vi "TrajectoryGenerate_Make_Quintic.vi"(8 "traj_config":T6 {"End Velocity" format="%20.4f"; "StartVelocity" format="%20.4f"; "Max Acceleration" format="%20.4f"; "MaxVelocity" format="%20.4f"}, 11 "waypointPOSE":T1[](array[typedef]) {"ROTATION"."SIN" format="%13.4f"; "ROTATION"."COS" format="%13.4f"; "ROTATION"."VALUE" format="%13.4f"; "TRANSLATION"."Y" format="%14.3f"; "TRANSLATION"."X" format="%14.3f"}) -> (0 "error out":errorcluster, 3 "TRAJECTORY":T4 {"States"."POSE"."ROTATION"."SIN" format="%13.4f"; "States"."POSE"."ROTATION"."COS" format="%13.4f"; "States"."POSE"."ROTATION"."VALUE" format="%13.4f"; "States"."POSE"."TRANSLATION"."Y" format="%14.3f"; "States"."POSE"."TRANSLATION"."X" format="%14.3f"; "TotalTImeSecs" format="%20.3f"})   [LabVIEW 2019, in "Trajectory_Library.lvlib"]
doc: "Generates a trajectory from the given waypoints and config. This method uses quintic hermite splines -- therefore, all points must be represented by Pose2d objects. Continuous curvature is guaranteed in this method.\n\nParameters:\n - WaypointPose - Array of waypoints (Pose).\n - Trajectory Config - The configuration for the trajectory.\n\nReturns:\n - Trajectory -- Created trajectory data structure\n - Error Out - Returned error cluster"
uses:
  Trajectory_Library.lvlib
  TypeDef/TRANSLATION2D.ctl
  TypeDef/ROTATION2D.ctl
  TypeDef/POSE2D.ctl
  TypeDef/POSEwCURVATURE.ctl
  TypeDef/TRAJ_STATE.ctl
  TypeDef/TRAJECTORY.ctl
  TypeDef/TRAJ_CONFIG.ctl
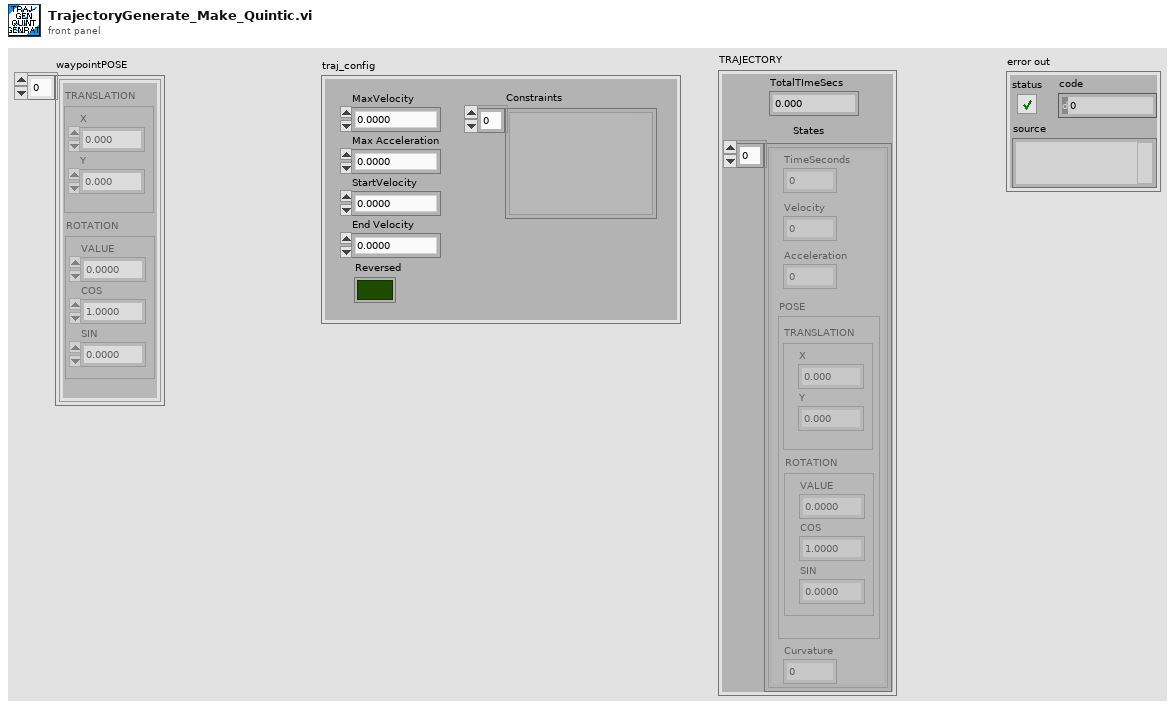
[diagram p1: front panel]
types:
  T1 = typedef "Trajectory_Library.lvlib/POSE2D.ctl" = cluster{"TRANSLATION":T2, "ROTATION":T3}
  T2 = typedef "Trajectory_Library.lvlib/TRANSLATION2D.ctl" = cluster{"X":dbl, "Y":dbl}
  T3 = typedef "Trajectory_Library.lvlib/ROTATION2D.ctl" = cluster{"VALUE":dbl, "COS":dbl, "SIN":dbl}
  T4 = typedef "Trajectory_Library.lvlib/TRAJECTORY.ctl" = cluster{"TotalTImeSecs":dbl, "States":T5[]}
  T5 = typedef "Trajectory_Library.lvlib/TRAJ_STATE.ctl" = cluster{"TimeSeconds":dbl, "Velocity":dbl, "Acceleration":dbl, "POSE":T1, "Curvature":dbl}
  T6 = typedef "Trajectory_Library.lvlib/TRAJ_CONFIG.ctl" = cluster{"MaxVelocity":dbl, "Max Acceleration":dbl, "StartVelocity":dbl, "End Velocity":dbl, "Reversed":bool, "Constraints":variant[]}
  T7 = typedef "WPILib_Math.lvlib/ROTATION2D.ctl" = cluster{"VALUE":dbl, "COS":dbl, "SIN":dbl}
  T8 = typedef "WPILib_Math.lvlib/TRANSLATION2D.ctl" = cluster{"X":dbl, "Y":dbl}
  T9 = typedef "WPILib_Math.lvlib/TRANSFORM2D.ctl" = cluster{"TRANSLATION":T8, "ROTATION":T7, "xF":bool}
  T10 = typedef "WPILib_Math.lvlib/POSE2D.ctl" = cluster{"TRANSLATION":T8, "ROTATION":T7}
  T11 = typedef "WPILib_Math.lvlib/SPLINE.ctl" = cluster{"Degree":i32, "Coefficients":T12}
  T12 = typedef "NI_Matrix.lvlib/RealMatrix.ctl" = dbl[][]
  T13 = typedef "Trajectory_Library.lvlib/POSEwCURVATURE.ctl" = cluster{"CURVATURE":dbl, "POSE":T1}
  T14 = typedef "WPILib_Math.lvlib/POSEwCURVATURE.ctl" = cluster{"CURVATURE":dbl, "POSE":T10}
  T15 = typedef "WPILib_Math.lvlib/TRAJECTORY.ctl" = cluster{"TotalTImeSecs":dbl, "States":T16[]}
  T16 = typedef "WPILib_Math.lvlib/TRAJ_STATE.ctl" = cluster{"TimeSeconds":dbl, "Velocity":dbl, "Acceleration":dbl, "POSE":T10, "Curvature":dbl}
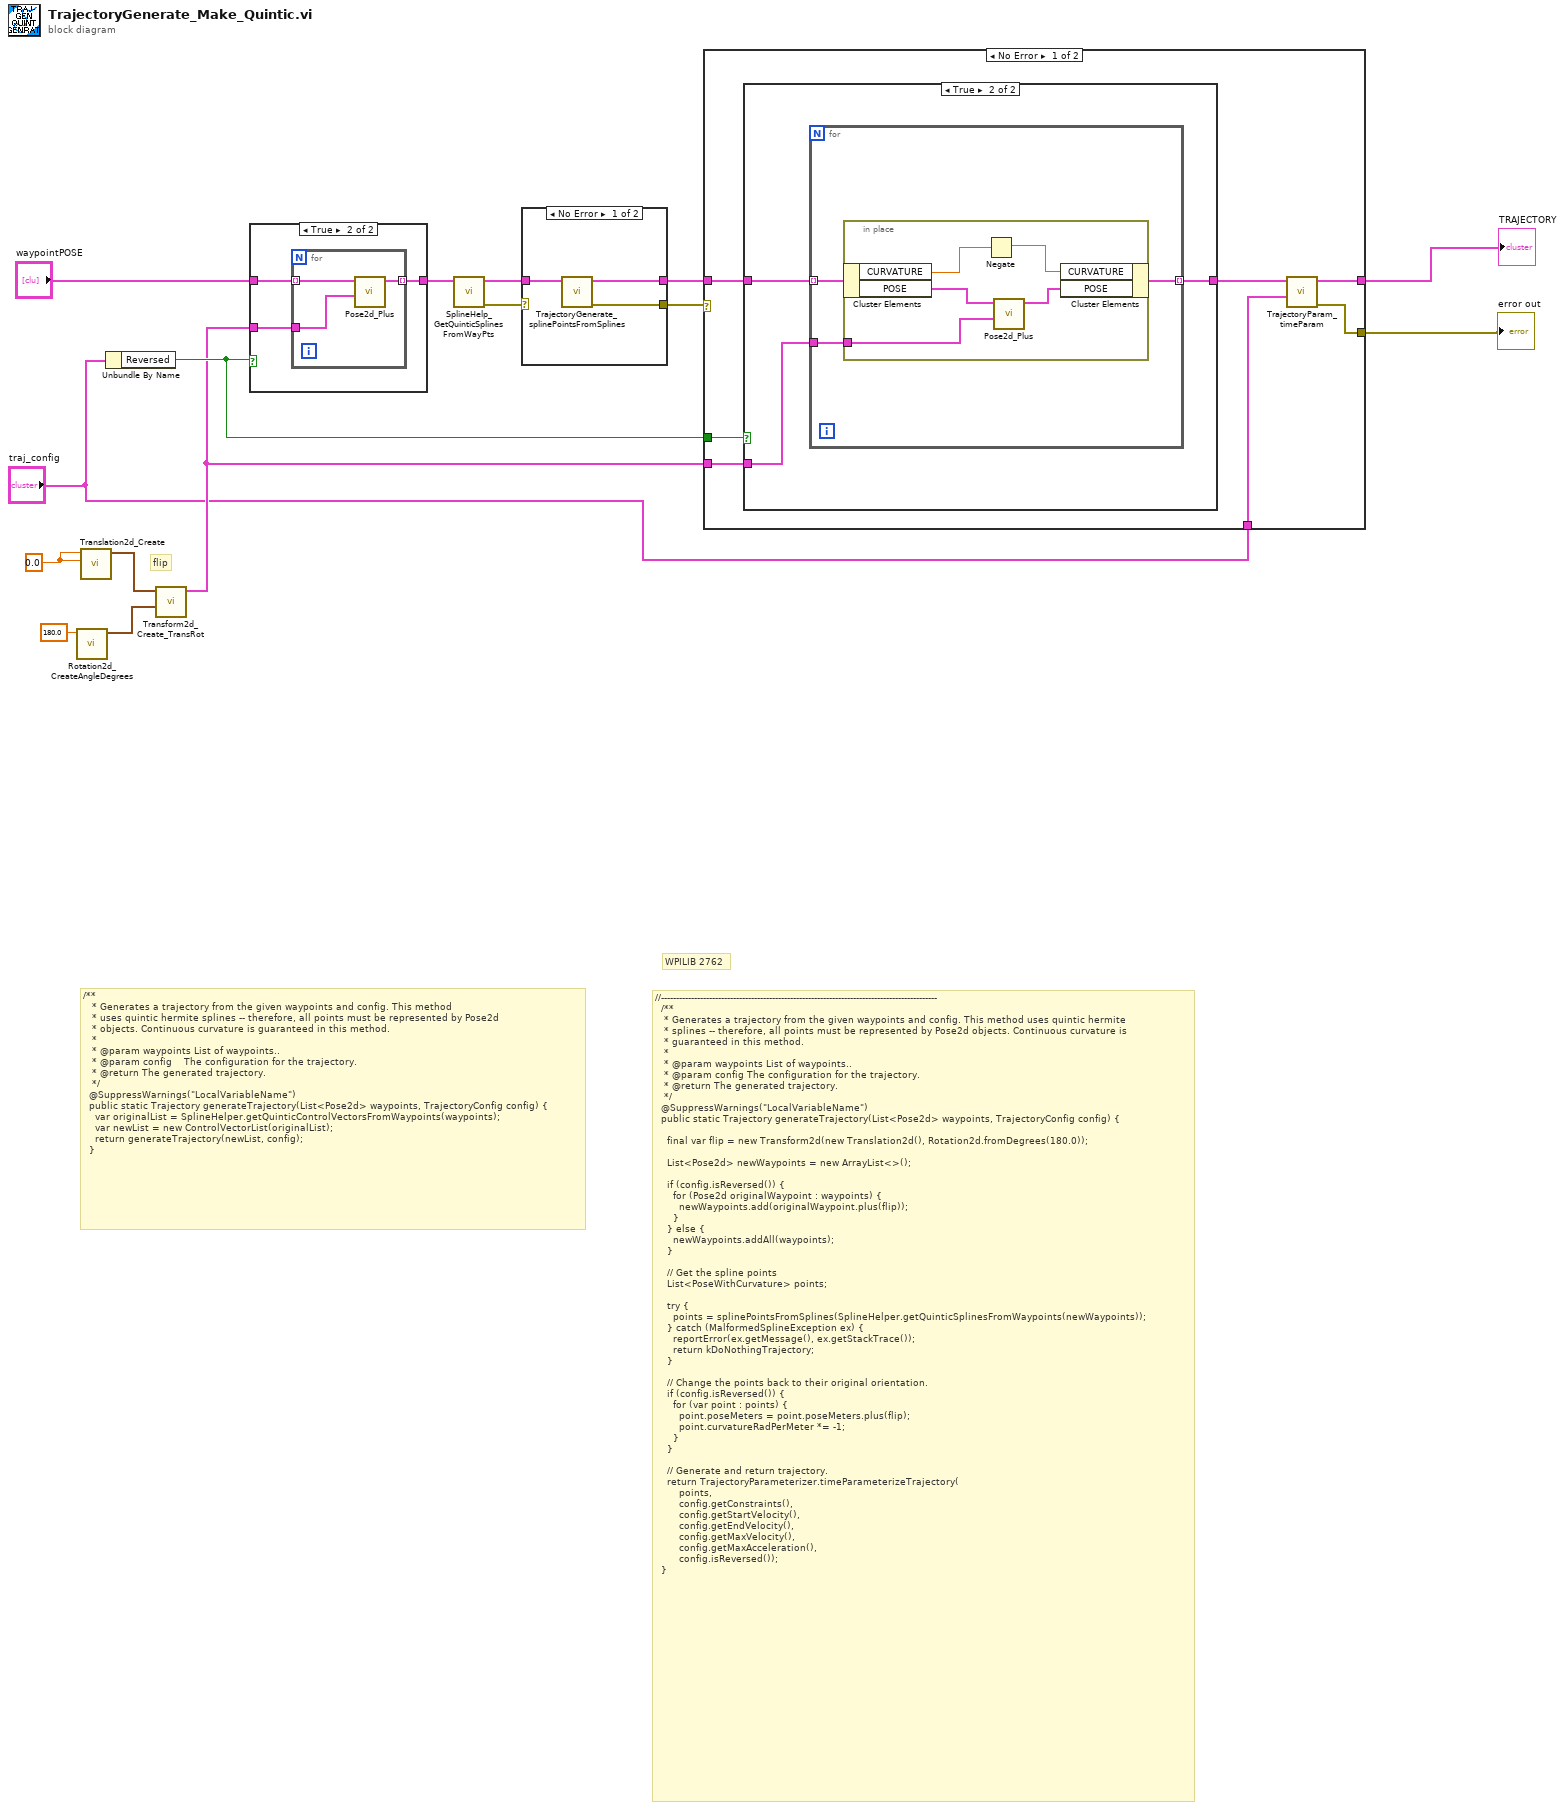
[diagram p0: block diagram]
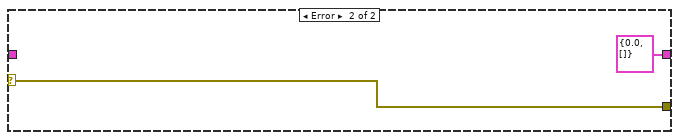
[diagram p3: hidden frame]
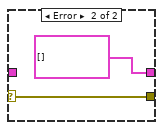
[diagram p4: hidden frame]
diagram:
  w13 = 0.0 ("X")
  # "flip"
  # "WPILIB 2762"
  # "//--------------------------------------------------------------------------------------------\n  /**\n   * Generates a trajectory from the given waypoints and config. This method uses quintic hermite\n   * splines -- therefore, all points must be represented by Pose2d objects. Continuous curvature is\n   * guaranteed in this method.\n   *\n   * @param waypoints List of waypoints..\n   * @param config The configuration for the trajectory.\n   * @return The generated trajectory.\n   */\n  @SuppressWarnings(\"LocalVariableName\")\n  public static Trajectory generateTrajectory(List<Pose2d> waypoints, TrajectoryConfig config) {\n\n    final var flip = new Transform2d(new Translation2d(), Rotation2d.fromDegrees(180.0));\n\n    List<Pose2d> newWaypoints = new ArrayList<>();\n\n    if (config.isReversed()) {\n      for (Pose2d originalWaypoint : waypoints) {\n        newWaypoints.add(originalWaypoint.plus(flip));\n      }\n    } else {\n      newWaypoints.addAll(waypoints);\n    }\n\n    // Get the spline points\n    List<PoseWithCurvature> points;\n\n    try {\n      points = splinePointsFromSplines(SplineHelper.getQuinticSplinesFromWaypoints(newWaypoints));\n    } catch (MalformedSplineException ex) {\n      reportError(ex.getMessage(), ex.getStackTrace());\n      return kDoNothingTrajectory;\n    }\n\n    // Change the points back to their original orientation.\n    if (config.isReversed()) {\n      for (var point : points) {\n        point.poseMeters = point.poseMeters.plus(flip);\n        point.curvatureRadPerMeter *= -1;\n      }\n    }\n\n    // Generate and return trajectory.\n    return TrajectoryParameterizer.timeParameterizeTrajectory(\n        points,\n        config.getConstraints(),\n        config.getStartVelocity(),\n        config.getEndVelocity(),\n        config.getMaxVelocity(),\n        config.getMaxAcceleration(),\n        config.isReversed());\n  }"
  # "/**\n   * Generates a trajectory from the given waypoints and config. This method\n   * uses quintic hermite splines -- therefore, all points must be represented by Pose2d\n   * objects. Continuous curvature is guaranteed in this method.\n   *\n   * @param waypoints List of waypoints..\n   * @param config    The configuration for the trajectory.\n   * @return The generated trajectory.\n   */\n  @SuppressWarnings(\"LocalVariableName\")\n  public static Trajectory generateTrajectory(List<Pose2d> waypoints, TrajectoryConfig config) {\n    var originalList = SplineHelper.getQuinticControlVectorsFromWaypoints(waypoints);\n    var newList = new ControlVectorList(originalList);\n    return generateTrajectory(newList, config);\n  }"
  n1 = call "Rotation2d_CreateAngleDegrees.vi"("Angle_Degrees"=180.0) -> ("ROTATION"=w15:T7)  [unwired: 10 in]
  n2 = call "Translation2d_Create.vi"("Y"=w13, "X"=w13) -> ("TRANSLATION"=w12:T8)  [unwired: 9 in]
  n3 = Unbundle By Name("traj_config") -> ("Reversed"=w6:bool)
  n4 = call "Transform2d_Create_TransRot.vi"("ROTATION"=w15, "TRANSLATION"=w12) -> ("TRANSFORM"=w4:T9)  [unwired: 9 in]
  n5 = case shown="True" w6 {
    tunnel: "waypointPOSE" -> [w16 w19]
    tunnel: w4 -> [_ w18]
    tunnel: [w16 w17] -> w10
    frame False {
    }
    frame True {
      n6 = for {
        tunnel: w19 -> [w22] mode=indexing
        tunnel: w18 -> [w21]
        tunnel: [w20] -> w17 mode=indexing
        n7 = call "Pose2d_Plus.vi"("other TRANSFORM"=w21, "in POSE"=w22) -> ("out POSE"=w20:T10)  [unwired: 9 in]
      }
    }
  }
  n8 = call "SplineHelp_GetQuinticSplinesFromWayPts.vi"("WayPoints"=w10) -> ("out Error"=w9:errorcluster, "Splines"=w8:T11[])  [unwired: 9 in]
  n9 = case shown="No Error" w9 {
    selector: w9 -> [_ w27]
    tunnel: w8 -> [w25 _]
    tunnel: [w24 w27] -> w7
    tunnel: [w23 T13[] [] ("ArrayPoseWithCurvature")] -> w5
    frame No Error {
      n10 = call "TrajectoryGenerate_splinePointsFromSplines.vi"("inputSPLINE"=w25) -> ("error out"=w24:errorcluster, "ArrayPoseWithCurvature"=w23:T14[])  [unwired: 9 in]
    }
    frame Error {
    }
  }
  n11 = case shown="No Error" w7 {
    selector: w7 -> [_ w48]
    tunnel: w6 -> [w34 _]
    tunnel: w5 -> [w33 _]
    tunnel: w4 -> [w32 _]
    tunnel: "traj_config" -> [w30 _]
    tunnel: [w29 T4 {"TotalTImeSecs"=0.0, "States"=[]} ("TRAJECTORY")] -> w2
    tunnel: [w28 w48] -> w1
    frame No Error {
      n12 = case shown="True" w34 {
        tunnel: w33 -> [w35 w38]
        tunnel: w32 -> [_ w37]
        tunnel: [w35 w36] -> w31
        frame False {
        }
        frame True {
          n13 = for {
            tunnel: w38 -> [w41] mode=indexing
            tunnel: w37 -> [w40]
            tunnel: [w39] -> w36 mode=indexing
            n14 = in-place {
              in-place-border: w40 -> [w42]
              n15 = in-place-cluster #1(w41) -> ("CURVATURE"=w46:dbl, "POSE"=w45:T1)
              n16 = Negate(x=w46) -> (-x=w43:dbl)
              n17 = call "Pose2d_Plus.vi"("other TRANSFORM"=w42, "in POSE"=w45) -> ("out POSE"=w44:T10)  [unwired: 9 in]
              n18 = in-place-cluster #1("CURVATURE"=w43, "POSE"=w44) -> (w39:T13)
            }
          }
        }
      }
      n19 = call "TrajectoryParam_timeParam.vi"("TRAJECTORY_CONFIG"=w30, "points"=w31) -> ("error out"=w28:errorcluster, "TRAJECTORY"=w29:T15)  [unwired: 8 in]
    }
    frame Error {
    }
  }
  "TRAJECTORY" <- w2
  "error out" <- w1
